vi "create_scan_steps_MR.vi"(7 "number of steps":u32, 9 "step":i32, 10 "stop":i32, 11 "start":i32) -> (1 "array length":i32, 3 "single steps":i32[](array[numeric]))   [LabVIEW 2015]
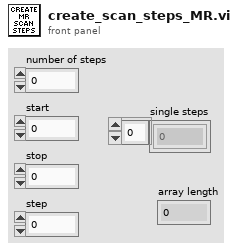
[diagram p1: front panel]
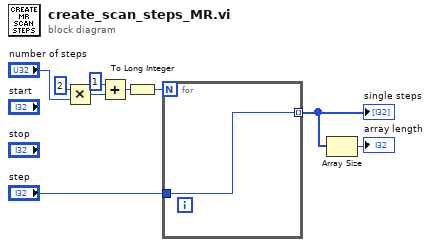
[diagram p0: block diagram]
diagram:
  n1 = Multiply(x=u32 2, y="number of steps") -> (x*y=w5:u32)
  n2 = Add(x=u32 1, y=w5) -> (x+y=w1:u32)
  n3 = To Long Integer(number=w1) -> (32bit integer=w6:i32)
  n4 = for {
    N: w6 -> [_]
    tunnel: "step" -> [w10]
    tunnel: [w10] -> w8 mode=indexing
  }
  "single steps" <- w8
  n5 = Array Size(array=w8) -> (size(s)=→"array length":i32)
